vi "Set Font.vi"(8 "error in":errorcluster, 10 "Font.lvclass":refnum<class "Font.lvclass">, 11 "View in":refnum<class "Cell View.lvclass">) -> (0 "error out":errorcluster, 3 "View out":refnum<class "Cell View.lvclass">)   [LabVIEW 2024, in "Cell View.lvclass"]
uses:
  Cell View.lvclass
  Font/Font.lvclass
  Cell View.lvclass/Cell View.ctl
  Font/Font.lvclass/Font.ctl
  D:/git/Sourcegrid-LabVIEW/dll/SourceGrid.dll
  dll/SourceGrid.dll
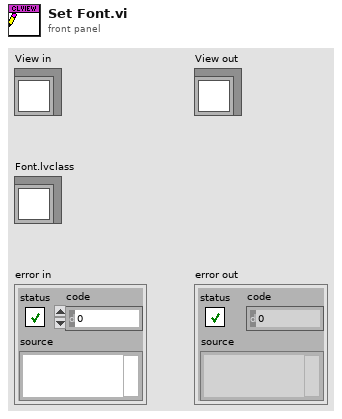
[diagram p1: front panel]
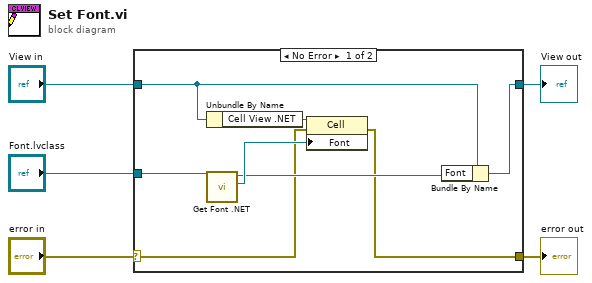
[diagram p0: block diagram]
diagram:
  n1 = case shown="No Error" "error in" {
    selector: "error in" -> [w7 w14]
    tunnel: [w6 w14] -> w4
    tunnel: [w13 w15] -> w2
    tunnel: "View in" -> [w12 w15]
    tunnel: "Font.lvclass" -> [w10 _]
    frame No Error {
      n2 = Unbundle By Name(w12) -> ("Cell View .NET"=w11:refnum<k24>)
      n3 = call "Get Font .NET.vi"("Font in"=w10) -> ("Font .NET"=w9:refnum<k24>, "Font out"=w8:refnum<class "Font.lvclass">)  [unwired: 9 in]
      n4 = property class="Cell"(reference=w11, error in=w7, "Font"=w9) -> (error out=w6:errorcluster)  [unwired: 1 out]
      n5 = Bundle By Name(cluster=w12, "Font"=w8) -> (w13:refnum<class "Cell View.lvclass">)
    }
    frame Error {
    }
  }
  "error out" <- w4
  "View out" <- w2
